vi "Read Results.vi"(11 "Job in":refnum<class "Job.lvclass">) -> (2 "Results":T1 {"Status" items=["Service Error"=504, "Abort"=503, "Fail"=500, "Pass"=200]})   [LabVIEW 2014, in "Job.lvclass"]
uses:
  Job.lvclass
  Controls/Job Results - STYP.ctl
  Job.lvclass/Job.ctl
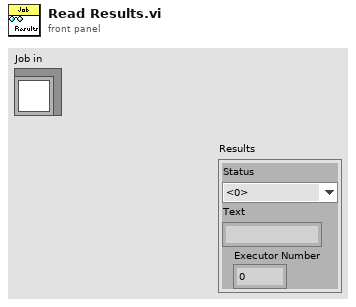
[diagram p1: front panel]
types:
  T1 = typedef "Job Results - STYP.ctl" = cluster{"Status":u16, "Text":string, "Executor Number":i32}
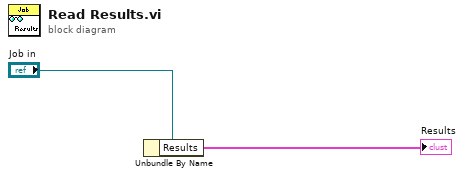
[diagram p0: block diagram]
diagram:
  n1 = Unbundle By Name("Job in") -> ("Results"=→"Results":T1)
